vi "Telemtery Main.vi"(8 "error IN":errorcluster, 11 "Aircraft Index":u8) -> ()   [LabVIEW 2014]
uses:
  Application Support/Stop Button/SubVI/Get Stop Button Status.vi
  Aircraft Information/Sub VI/Get Aircraft Information.vi
  Ground Station to Aircraft Coms/SubVI/Aircraft Data Router/SubVI/Queue References/SubVI/Get Aircraft RX Queue String.vi
  <vilib>/Instr/_visa.llb/VISA Flush IO Buffer Mask.ctl
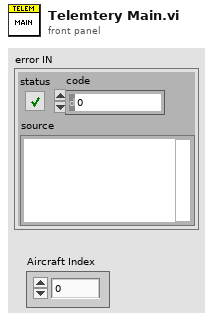
[diagram p1: front panel]
types:
  T1 = typedef "Drone Information.ctl" = cluster{"Aircraft ID":u8, "Tag ID":string, "System Status":string, "Base Mode":T2, "Armed/Disarmed":bool, "Battery Voltage":dbl, "Control Mode":T3, "Initialisation":u8, "Coms with aircraft good":bool, "Mode":string, "Mission Uploaded":bool}
  T2 = typedef "Base Mode.ctl" = cluster{"Custom Mode":bool, "Test Enabled":bool, "Autonomous Mode":bool, "Guided Mode":bool, "Stabilization Enabled":bool, "HIL Enabled":bool, "Manual Mode":bool, "Arm":bool}
  T3 = typedef "Aircraft Mode.ctl" = enum16{"Loiter", "Stabalise", "Failsafe", "Emergency Stop"}
  T4 = typedef "Telemetry Connection Type.ctl" = enum16{"Serial", "UDP", "TCP"}
  T5 = typedef "VISA Flush IO Buffer Mask.ctl" = u16
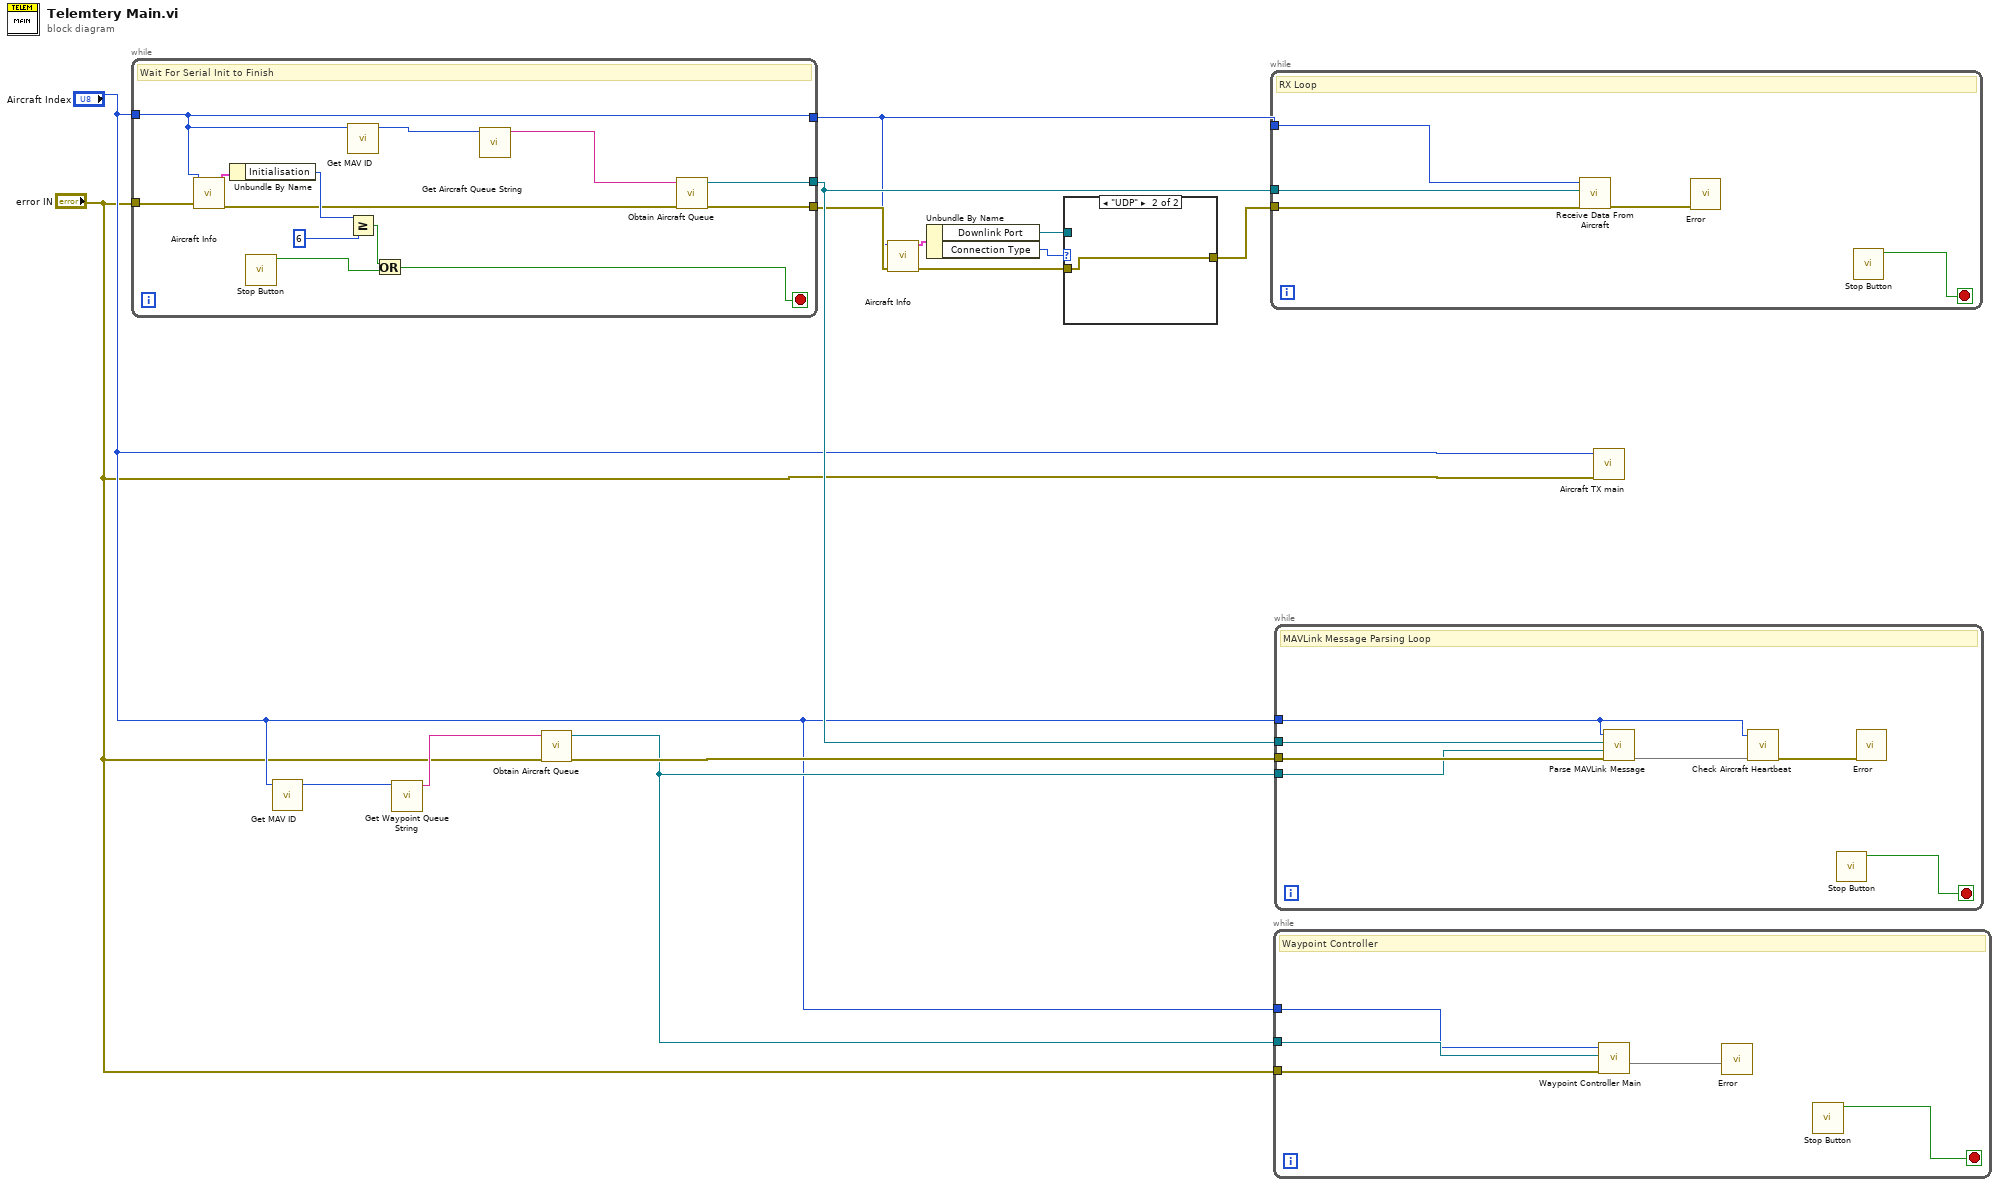
[diagram p0: block diagram]
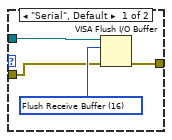
[diagram p2: hidden frame]
diagram:
  n1 = while {
    tunnel: "error IN" -> [w23]
    tunnel: [w18] -> w8
    tunnel: "Aircraft Index" -> [w16]
    tunnel: [w16] -> w7
    tunnel: [w17] -> w14
    stop <- w27 stop-if-true
    # "Wait For Serial Init to Finish"
    n2 = call-poly "Aircraft Info.vi"("Error In"=w23, "Aircraft ID"=w16) -> ("Error Out"=w19:errorcluster, "Aircraft Information Out"=w22:T1)  [unwired: 8 in]
    n3 = Unbundle By Name(w22) -> ("Initialisation"=w21:u8)
    n4 = call-poly "Stop Button.vi"() -> ("Stop ButtonOut"=w24:bool)  [unwired: 10 in, 1 out]
    n5 = call "Get MAV ID.vi"("Aircraft Index"=w16) -> ("Aircraft ID"=w15:u8)  [unwired: 9 in, 1 out]
    n6 = Greater Or Equal?(x=w21, y=u8 6) -> (x >= y?=w25:bool)
    n7 = Or(x=w25, y=w24) -> (x .or. y?=w27:bool)
    n8 = call-poly "Get Aircraft Queue String.vi"("Aircraft ID"=w15) -> ("Aircraft Q Name"=w20:string)  [unwired: 9 in, 1 out]
    n9 = call "Obtain Aircraft Queue.vi"("error in (no error)"=w19, "Queue Name"=w20) -> ("error out"=w18:errorcluster, "queue out"=w17:refnum<queue>)  [unwired: 8 in]
  }
  n10 = call "Get MAV ID.vi"("Aircraft Index"="Aircraft Index") -> ("Aircraft ID"=w13:u8)  [unwired: 9 in, 1 out]
  n11 = call "Get Waypoint Queue String.vi"("Aircraft ID"=w13) -> ("Aircraft Q Name"=w11:string)  [unwired: 10 in]
  n12 = call "Obtain Aircraft Queue.vi"("error in (no error)"="error IN", "Queue Name"=w11) -> ("error out"=w12:errorcluster, "queue out"=w10:refnum<queue>)  [unwired: 8 in]
  n13 = call-poly "Aircraft Info.vi"("Error In"=w8, "Aircraft ID"=w7) -> ("Error Out"=w4:errorcluster, "Aircraft Information Out"=w5:T1)  [unwired: 8 in]
  n14 = Unbundle By Name(w5) -> ("Downlink Port"=w3:refnum<visa-resource-name>, "Connection Type"=w6:T4)
  n15 = case shown="\"UDP\"" w6 {
    tunnel: w4 -> [w29 w32]
    tunnel: w3 -> [w31 _]
    tunnel: [w28 w32] -> w2
    frame "Serial", Default {
      w30 = T5 16 items=["Flush Receive Buffer"=16, "Write Transmit Buffer to Device"=32, "Flush Receive Buffer (No I/O)"=64, "Flush Transmit Buffer"=128] ("Mask")
      n16 = VISA Flush I/O Buffer(VISA resource name=w31, mask (16)=w30, error in (no error)=w29) -> (error out=w28:errorcluster)  [unwired: 1 out]
    }
    frame "UDP" {
    }
  }
  n17 = while {
    tunnel: w2 -> [w37]
    tunnel: w7 -> [w35]
    tunnel: w14 -> [w33]
    stop <- w34 stop-if-true
    # "RX Loop"
    n18 = call "Receive Data From Aircraft.vi"("error in (no error)"=w37, 10:w33, 11:w35) -> ("error out"=w36:errorcluster)  [unwired: 8 in]
    n19 = call "Error.vi"("Error In"=w36) -> ()  [unwired: 10 in, 1 out]
    n20 = call-poly "Stop Button.vi"() -> ("Stop ButtonOut"=w34:bool)  [unwired: 10 in, 1 out]
  }
  n21 = while {
    tunnel: "error IN" -> [w41]
    tunnel: w10 -> [w40]
    tunnel: "Aircraft Index" -> [w39]
    stop <- w42 stop-if-true
    # "Waypoint Controller"
    n22 = call "Waypoint Controller Main.vi"(8:w41, 10:w40, "Instance Details"=w39) -> (0:w38)  [unwired: 8 in]
    n23 = call "Error.vi"("Error In"=w38) -> ()  [unwired: 10 in, 1 out]
    n24 = call-poly "Stop Button.vi"() -> ("Stop ButtonOut"=w42:bool)  [unwired: 10 in, 1 out]
  }
  n25 = while {
    tunnel: w12 -> [w49]
    tunnel: "Aircraft Index" -> [w46]
    tunnel: w14 -> [w44]
    tunnel: w10 -> [w43]
    stop <- w45 stop-if-true
    # "MAVLink Message Parsing Loop"
    n26 = call "Parse MAVLink Message.vi"(8:w49, 9:w43, 10:w44, "Instance Details"=w46) -> (0:w47)  [unwired: 7 in]
    n27 = call "Check Aircraft Heartbeat.vi"("error in (no error)"=w47, "Aircraft ID"=w46) -> ("Error Out"=w48:errorcluster)  [unwired: 9 in]
    n28 = call-poly "Stop Button.vi"() -> ("Stop ButtonOut"=w45:bool)  [unwired: 10 in, 1 out]
    n29 = call "Error.vi"("Error In"=w48) -> ()  [unwired: 10 in, 1 out]
  }
  n30 = call "Aircraft TX main.vi"(8:"error IN", "Instance Details"="Aircraft Index") -> ()  [unwired: 10 in]
